vi "EKF.vi"(6 "init":bool, 9 "Messrausch":dbl[](array[numeric]), 10 "input":T1, 11 "Measurements":T1=[324600.0, 6006600.0]) -> (3 "act filtered coord":T1=[324600.0, 6006600.0])   [LabVIEW 2019]
uses:
  coordinate.ctl
  <vilib>/Analysis/baseanly.llb/Real A x B.vi
  <vilib>/Analysis/baseanly.llb/A x Vector.vi
  <vilib>/Analysis/Matrix/Numeric/Subtract/Subtract - RM,RM.vi
  <vilib>/Analysis/7linalg.llb/Create Special Real Matrix.vi
  <vilib>/Analysis/Matrix/Numeric/Multiply/Multiply - RM,R.vi
  <vilib>/Analysis/NI_AALPro.lvlib
  <vilib>/Analysis/Matrix/NI_Matrix.lvlib
  <vilib>/Analysis/NI_AALBase.lvlib
panel:
  in  "Nr Measurements":i32=3
  in  "order":i32=3
  out "state k+1":T1
  # "Replace Fk-Vi for aktual Model"
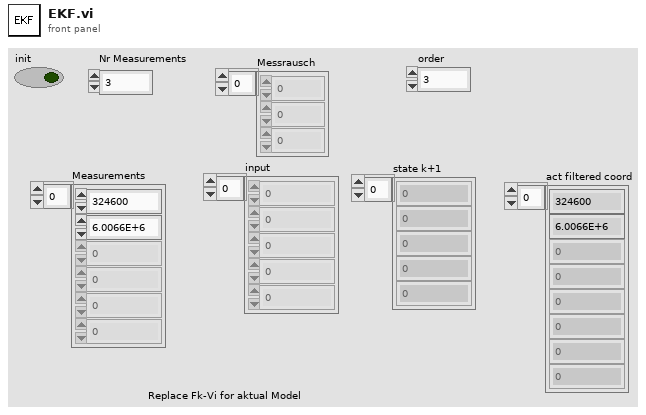
[diagram p1: front panel]
types:
  T1 = typedef "coordinate.ctl" = dbl[]
  T2 = typedef "NI_Matrix.lvlib/RealMatrix.ctl" = dbl[][]
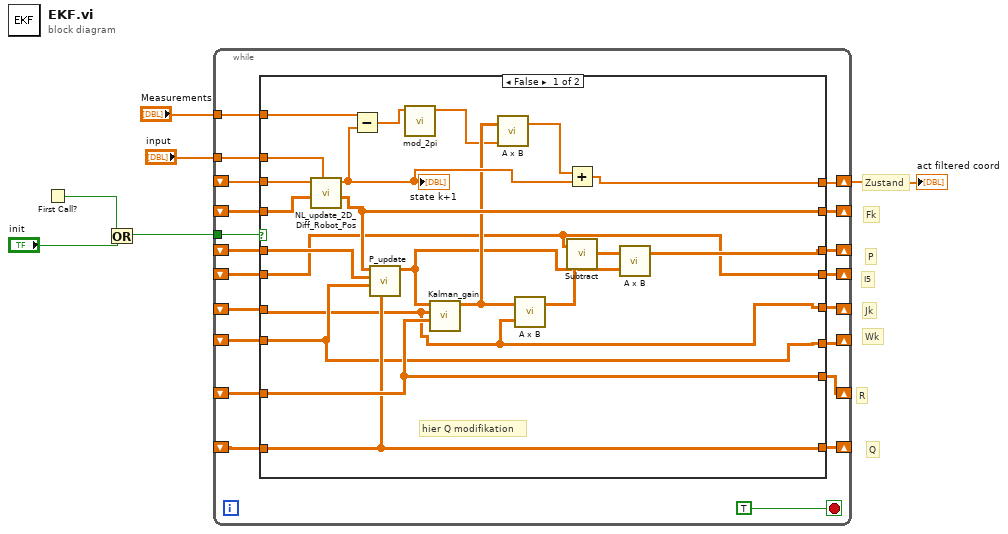
[diagram p0: block diagram]
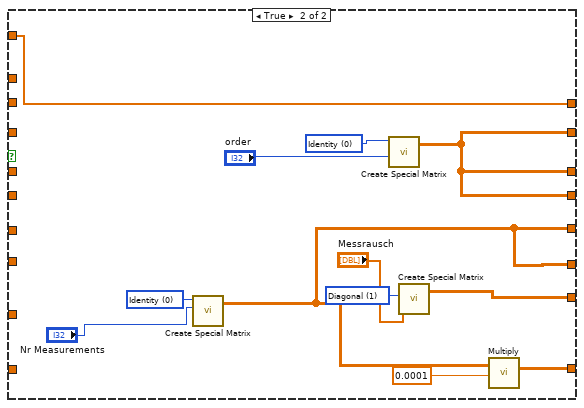
[diagram p2: hidden frame]
diagram:
  # "Wk"
  # "I5"
  # "Q"
  # "Jk"
  # "Fk"
  # "R"
  # "P"
  # "Zustand"
  n1 = First Call?() -> (First Call?: T/F=w2:bool)
  n2 = Or(x=w2, y="init") -> (x .or. y?=w3:bool)
  n3 = while {
    tunnel: w3 -> [w25]
    tunnel: "Measurements" -> [w24]
    shift-right: [w23] -> w4
    shift-left: _ -> [w20]
    shift-right: [w21] -> _
    shift-left: _ -> [w16]
    shift-right: [w22] -> _
    shift-left: _ -> [w12]
    shift-right: [w19] -> _
    shift-left: _ -> [w18]
    shift-right: [w17] -> _
    shift-left: _ -> [w15]
    shift-right: [w14] -> _
    shift-left: _ -> [w13]
    shift-right: [w11] -> _
    shift-left: _ -> [w10]
    shift-right: [w9] -> _
    shift-left: _ -> [w8]
    tunnel: "input" -> [w7]
    stop <- TRUE stop-if-true
    n4 = case shown="False" w25 {
      tunnel: w24 -> [w40 w59]
      tunnel: [w32 w59] -> w23
      tunnel: [w43 w55] -> w22
      tunnel: [w34 w54] -> w21
      tunnel: w20 -> [w47 _]
      tunnel: [w44 w54] -> w19
      tunnel: w18 -> [w46 _]
      tunnel: [w30 w50] -> w17
      tunnel: w16 -> [w45 _]
      tunnel: w15 -> [w30 _]
      tunnel: [w42 w53] -> w14
      tunnel: w13 -> [w42 _]
      tunnel: w12 -> [w43 _]
      tunnel: [w33 w54] -> w11
      tunnel: w10 -> [w33 _]
      tunnel: [w31 w50] -> w9
      tunnel: w8 -> [w31 _]
      tunnel: w7 -> [w29 _]
      frame False {
        # "hier Q modifikation"
        n5 = call "NL_update_2D_Diff_Robot_Pos.vi"("Input Delta s"=w29, "Fk"=w46, "state k"=w47) -> ("Fk+1"=w44:T2, "state k+1"=w41:T1)  [unwired: 7 in]
        "state k+1" <- w41
        n6 = Subtract(x=w40, y=w41) -> (x-y=w28:T1)
        n7 = call "P_update.vi"("Q"=w42, "Wk"=w31, "Pk-1"=w45, "Fk"=w44) -> ("Pk"=w35:T2)  [unwired: 7 in]
        n8 = call "mod_2pi.vi"("state k+1"=w28) -> ("state_mod2pi"=w27:T1)  [unwired: 10 in]
        n9 = call "Kalman_gain.vi"("R"=w43, "Jk"=w30, "Pk"=w35) -> ("K"=w38:T2)  [unwired: 8 in]
        n10 = call-poly <vilib>:"A x B.vi"("Vector"=w27, "A"=w38) -> ("A x Vector"=w39:dbl[])  [unwired: 1 out]
        n11 = call-poly <vilib>:"A x B.vi"("B"=w30, "A"=w38) -> ("A x B"=w37:T2)  [unwired: 1 out]
        n12 = Add(x=w39, y=w41) -> (x+y=w32:T1)
        n13 = call-poly <vilib>:"Subtract.vi"("Real Matrix B"=w37, "Real Matrix A"=w33) -> ("A - B"=w36:T2)
        n14 = call-poly <vilib>:"A x B.vi"("B"=w35, "A"=w36) -> ("A x B"=w34:T2)  [unwired: 1 out]
      }
      frame True {
        w49 = 1 items=["Identity", "Diagonal", "Toeplitz", "Vandermonde", "Companion", "Hankel", "Hadamard", "Wilkinson", "Hilbert", "Inverse Hilbert", "Rosser", "Pascal"] ("matrix type")
        w57 = 0 items=["Identity", "Diagonal", "Toeplitz", "Vandermonde", "Companion", "Hankel", "Hadamard", "Wilkinson", "Hilbert", "Inverse Hilbert", "Rosser", "Pascal"] ("matrix type")
        w58 = 0 items=["Identity", "Diagonal", "Toeplitz", "Vandermonde", "Companion", "Hankel", "Hadamard", "Wilkinson", "Hilbert", "Inverse Hilbert", "Rosser", "Pascal"] ("matrix type")
        n15 = call-poly <vilib>:"Create Special Matrix.vi"("matrix type"=w57, "matrix size"="Nr Measurements") -> ("Special Matrix"=w50:T2)  [unwired: 3 in, 1 out]
        n16 = call-poly <vilib>:"Create Special Matrix.vi"("matrix type"=w58, "matrix size"="order") -> ("Special Matrix"=w54:T2)  [unwired: 3 in, 1 out]
        n17 = call-poly <vilib>:"Create Special Matrix.vi"("matrix type"=w49, "Input Vector1"="Messrausch") -> ("Special Matrix"=w55:T2)  [unwired: 3 in, 1 out]
        n18 = call-poly <vilib>:"Multiply.vi"("Real Scalar c"=0.0001, "Real Matrix A"=w50) -> ("A * c"=w53:T2)
      }
    }
  }
  "act filtered coord" <- w4
